vi "initialise.vi"(8 "error in (no error)":errorcluster, 10 "writer buffer size":i32=100000 format="%.0e") -> (0 "error out":errorcluster, 2 "network streaming queues":T2, 3 "FPGA VI Reference Out":T1)   [LabVIEW 2010]
uses:
  network_streaming_queues_cluster.ctl
  type definitions/config_data_cluster.ctl
  type definitions/settings_cluster.ctl
  common_typedefs/channels_cluster.ctl
  type definitions/gate_cluster.ctl
  common_typedefs/gate_parameters_cluster.ctl
  FPGA_VI_reference.ctl
  <vilib>/userDefined/High Color/nirio_resource_hc.ctl
  type definitions/command_enum.ctl
  <vilib>/rvi/interface/nirviOpenFPGA/nirviOpenFPGA.xnode
  FPGA Bitfiles/PCIe-7842R_80MHz.lvbitx
  <vilib>/rvi/ClientSDK/nirviWhatTheDeviceIsDoing.ctl
  <vilib>/rvi/interface/nirviMethod/nirviMethod.xnode
  <vilib>/rvi/interface/nirviReadWriteControl/nirviReadWriteControl.xnode
  <vilib>/rvi/interface/common/niFpgaNodeNameForErrorReporting.ctl
  <vilib>/rvi/errors/niLvFpgaWhatHappensToTopLevelVI.ctl
  <vilib>/FPGAPlugInAG/PCIe-7842R/niLvFpga_Open_PCIe-7842R.vi
  <vilib>/rvi/interface/common/dynamic/niFpgaDynamicAddResources.vi
  <vilib>/Utility/error.llb/Error Cluster From Error Code.vi
  <vilib>/FPGAPlugInAG/Dynamic/niLvFpga_Reset_Dynamic.vi
  <vilib>/rvi/errors/niLvFpgaAdjustHostInterfaceError.vi
  NiFpgaLv.dll
panel:
  out "hifo box version":i32
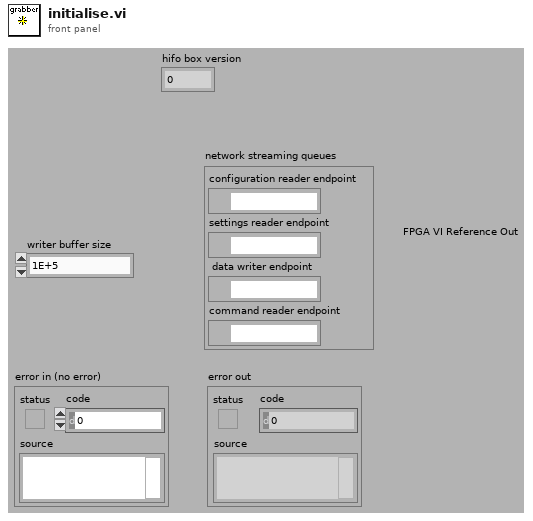
[diagram p1: front panel]
types:
  T1 = typedef "FPGA_VI_reference.ctl" = refnum<k20>
  T2 = typedef "network_streaming_queues_cluster.ctl" = cluster{"configuration reader endpoint":refnum<k21>, "settings reader endpoint":refnum<k21>, "data writer endpoint":refnum<k21>, "command reader endpoint":refnum<k21>}
  T3 = enum32{"Invalid", "Standard", "Closed", "Hidden", "Minimized", "Maximized"}
  T4 = typedef "config_data_cluster.ctl" = cluster{"bit file":string, "hifo box version":i32, "ADC clock phase":i32}
  T5 = typedef "settings_cluster.ctl" = cluster{"number of pixels":i64, "pixel frequency (Hz)":dbl, "pixel values cluster":T6, "triggered?":bool, "triggered flag valid?":bool, "gates":T7[]}
  T6 = typedef "channels_cluster.ctl" = cluster{"channel 0":u32, "channel 1":u32, "channel 2":u32, "channel 3":u32}
  T7 = typedef "gate_cluster.ctl" = cluster{"index":i32, "parameters":T8}
  T8 = typedef "gate_parameters_cluster.ctl" = cluster{"offset":i64, "pulsing":i64, "not pulsing":i64, "cycles per pulse":i64, "repetitions":i64}
  T9 = typedef "nirio_resource_hc.ctl" = tag
  T10 = typedef "command_enum.ctl" = enum16{"NULL", "update", "start", "stop", "reset", "shut-down"}
  T11 = typedef "nirviWhatTheDeviceIsDoing.ctl" = enum32{"nothing", "something other than LabVIEW FPGA", "FPGA interface", "interactive", "emulation"}
  T12 = typedef "niFpgaNodeNameForErrorReporting.ctl" = enum16{"Open FPGA VI Reference", "Read/Write Control", "Invoke Method: Abort", "Invoke Method: Acknowledge IRQ", "Invoke Method: Download", "Invoke Method: FIFO.Configure", "Invoke Method: FIFO.Read", "Invoke Method: FIFO.Start", "Invoke Method: FIFO.Stop", "Invoke Method: FIFO.Write", "Invoke Method: Reset", "Invoke Method: Run", "Invoke Method: Wait on IRQ", "Close FPGA VI Reference"}
  T13 = typedef "niLvFpgaWhatHappensToTopLevelVI.ctl" = enum16{"top level VI scripted behind XNode", "top level VI inlined behind XNode"}
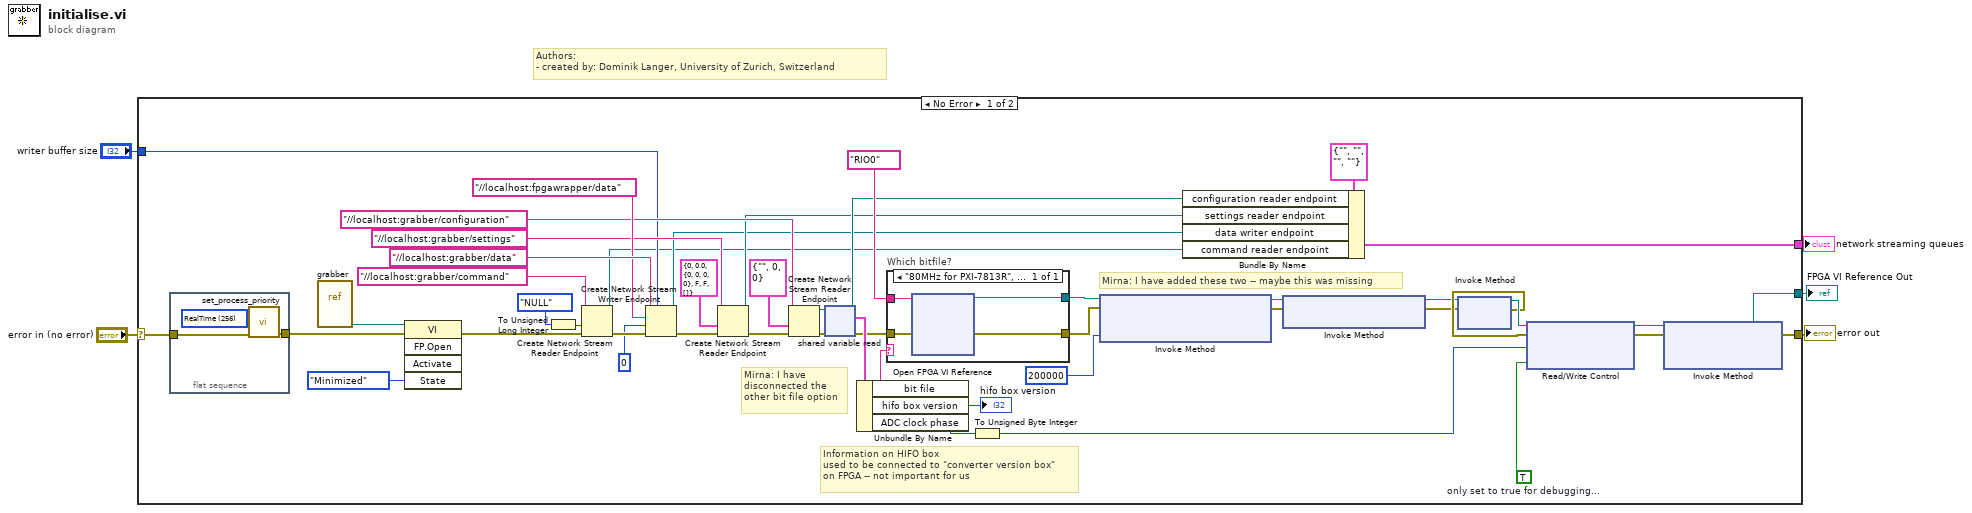
[diagram p0: block diagram]
diagram:
  # "Authors: \n- created by: Dominik Langer, University of Zurich, Switzerland"
  n1 = case shown="No Error" "error in (no error)" {
    selector: "error in (no error)" -> [w28 w267]
    tunnel: [w27 w267] -> w4
    tunnel: "writer buffer size" -> [w26 _]
    tunnel: [w20 _] -> w2
    tunnel: [w19 _] -> w1
    frame No Error {
      w6 = TRUE  # only set to true for debugging...
      # "Information on HIFO box\nused to be connected to \"converter version box\"\non FPGA -- not important for us"
      # "Mirna: I have \ndisconnected the\nother bit file option"
      # "Mirna: I have added these two -- maybe this was missing"
      n2 = flat-sequence {
        tunnel: [w265] -> w17
        tunnel: w28 -> [w264]
        frame #0 {
          w266 = 256 items=["Normal"=32, "Idle"=64, "High"=128, "RealTime"=256, "BelowNormal"=16384, "AboveNormal"=32768] ("PriorityClass")
          n3 = call "set_process_priority.vi"("error in (no error)"=w264, "PriorityClass"=w266) -> ("error out"=w265:errorcluster)  [unwired: 9 in]
        }
      }
      n4 = vi-ref "grabber.vi"() -> (w18:refnum<vi>)
      n5 = invoke class="VI" method="FP.Open"(reference=w18, error in=w17, "State"=T3."Minimized") -> (error out=w16:errorcluster)  [unwired: 2 in, 4 out]
      n6 = To Unsigned Long Integer(number=command_enum."NULL" ("command")) -> (unsigned 32bit integer=w52:u32)
      n7 = Create Network Stream Reader Endpoint(8:w16, 9:w52, 11:"//localhost:grabber/command" ("writer name")) -> (0:w34:errorcluster, 3:w21:refnum<k21>)  [unwired: 3 in]
      n8 = Create Network Stream Writer Endpoint(7:w26, 8:w34, 9:u64 0, 10:"//localhost:fpgawrapper/data" ("reader url"), 11:"//localhost:grabber/data" ("writer name")) -> (0:w33:errorcluster, 3:w22:refnum<k21>)  [unwired: 1 in]
      n9 = Create Network Stream Reader Endpoint(8:w33, 9:T5 {"number of pixels"=0, "pixel frequency (Hz)"=0.0, "pixel values cluster"={"channel 0"=0, "channel 1"=0, "channel 2"=0, "channel 3"=0}, "triggered?"=FALSE, "triggered flag valid?"=FALSE, "gates"=[]} ("settings"), 11:"//localhost:grabber/settings" ("reader url")) -> (0:w36:errorcluster, 3:w23:refnum<k21>)  [unwired: 3 in]
      n10 = Create Network Stream Reader Endpoint(8:w36, 9:T4 {"bit file"="", "hifo box version"=0, "ADC clock phase"=0} ("config data"), 11:"//localhost:grabber/configuration" ("reader url")) -> (0:w48:errorcluster, 3:w47:refnum<k21>)  [unwired: 3 in]
      n11 = shared-variable-read(w47, w48) -> (w24:refnum<k21>, w40:errorcluster, w42:T4)  [unwired: 1 in, 1 out]
      n12 = Unbundle By Name(w42) -> ("bit file"=w39:string, "hifo box version"=→"hifo box version":i32, "ADC clock phase"=w38:i32)
      n13 = case "Which bitfile?" shown="\"80MHz for PXI-7813R\", Default" w39 {
        tunnel: w40 -> [w103]
        tunnel: [w102] -> w11
        tunnel: T9 "RIO0" ("resource name") -> [w101]
        tunnel: [w100] -> w12
        frame "80MHz for PXI-7813R", Default {
          n14 = xnode "Open FPGA VI Reference"("error in"=w103, "resource name"=w101) -> ("FPGA VI Reference Out"=w100:refnum<k20>, "error out"=w102:errorcluster)
        }
      }
      n15 = To Unsigned Byte Integer(number=w38) -> (unsigned 8bit integer=w7:u8)
      n16 = xnode "Invoke Method"("FPGA VI Reference In"=w12, "error in"=w11, "Depth"=u32 200000) -> ("FPGA VI Reference Out"=w15:refnum<k20>, "error out"=w14:errorcluster)
      n17 = Bundle By Name(cluster=T2 {"configuration reader endpoint"="", "settings reader endpoint"="", "data writer endpoint"="", "command reader endpoint"=""} ("network streaming queues"), "configuration reader endpoint"=w24, "settings reader endpoint"=w23, "data writer endpoint"=w22, "command reader endpoint"=w21) -> (w20:T2)
      n18 = xnode "Invoke Method"("FPGA VI Reference In"=w15, "error in"=w14) -> ("FPGA VI Reference Out"=w10:refnum<k20>, "error out"=w9:errorcluster)
      n19 = xnode "Invoke Method"("FPGA VI Reference In"=w10, "error in"=w9) -> ("FPGA VI Reference Out"=w46:refnum<k20>, "error out"=w45:errorcluster)
      n20 = xnode "Read/Write Control"("FPGA VI Reference In"=w46, "error in"=w45, "ADC clock phase"=w7, "clamp first pixel?"=w6) -> ("FPGA VI Reference Out"=w43:refnum<k20>, "error out"=w44:errorcluster)
      n21 = xnode "Invoke Method"("FPGA VI Reference In"=w43, "error in"=w44) -> ("FPGA VI Reference Out"=w19:refnum<k20>, "error out"=w27:errorcluster)  [unwired: 1 in]
    }
    frame Error {
    }
  }
  "error out" <- w4
  "network streaming queues" <- w2
  "FPGA VI Reference Out" <- w1
